vi "Get Rooms.vi"(8 "error in (no error)":errorcluster, 11 "Room-API in":refnum<class "Room-API.lvclass">) -> (0 "error out":errorcluster, 2 "roomIds":string[](array[string]), 3 "Room-API out":refnum<class "Room-API.lvclass">)   [LabVIEW 2020, in "Room-API.lvclass"]
uses:
  Room-API.lvclass
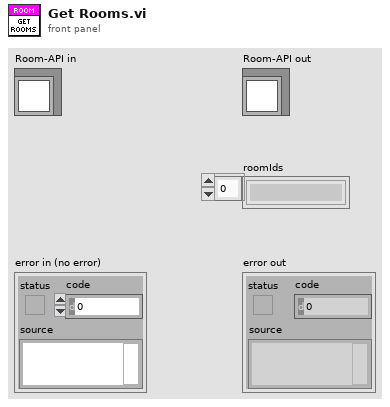
[diagram p1: front panel]
types:
  T1 = typedef "Room-API.lvclass/Single Room.ctl" = cluster{"name":string, "temperature_humidity":string[], "bond":string[], "hue":string[]}
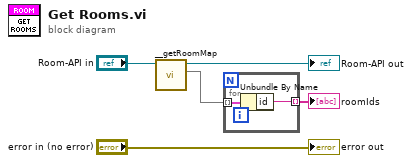
[diagram p0: block diagram]
diagram:
  n1 = call "__getRoomMap.vi"("Room-API in"="Room-API in") -> ("room_map"=w3:map{string, T1}, "Room-API out"=→"Room-API out":refnum<class "Room-API.lvclass">)  [unwired: 9 in]
  n2 = for {
    tunnel: w3 -> [w7] mode=indexing
    tunnel: [w6] -> w2 mode=indexing
    n3 = Unbundle By Name(w7) -> ("id"=w6:string)
  }
  "roomIds" <- w2
  "error out" <- "error in (no error)"
